vi "HTML Hierarhy Open Branch.vi"(8 "error in":errorcluster, 9 "checked":bool, 10 "id":string, 11 "label":string) -> (0 "error out":errorcluster)   [LabVIEW 2014, in "lvprj2html.lvlib"]
uses:
  lvprj2html.lvlib
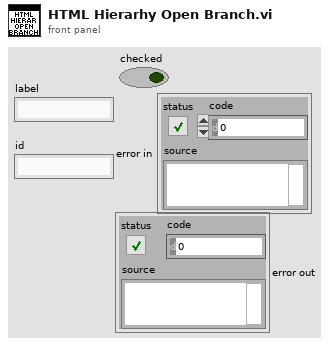
[diagram p1: front panel]
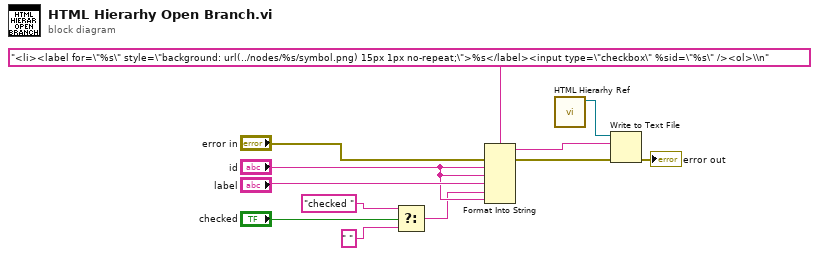
[diagram p0: block diagram]
diagram:
  n1 = Select(t="checked " ("label"), s="checked", f=" " ("label")) -> (s? t:f=w6:string)
  n2 = Format Into String(format string="<li><label for=\"%s\" style=\"background: url(../nodes/%s/symbol.png) 15px 1px no-repeat;\">%s</label><input type=\"checkbox\" %sid=\"%s\" /><ol>\\n" ("text"), error in="error in", "id", "id", "label", w6, "id") -> (resulting string=w8:string, error out=w2:errorcluster)  [unwired: 1 in]
  n3 = call "HTML Hierarhy Ref.vi"() -> ("Byte Stream File out"=w12:refnum<file>)  [unwired: 11 in]
  n4 = Write to Text File(file (use dialog)=w12, text=w8, error in=w2) -> (error out=→"error out":errorcluster)  [unwired: 1 in, 2 out]
